vi "ADC_Driver.vi"() -> ()   [LabVIEW 2020]
uses:
  <vilib>/numeric/Random Number (Range) DBL.vi
panel:
  out "Digital Waveform Graph":digitaldata(graph)
  out "Output Waveform":digitaldata
  out "x-y":u8[](array[numeric])
  out "Waveform Graph":u8[](graph)
  out "Unsigned Byte Array":u8[](array[numeric])
  out "Binary String":string
  out "Digital before U8":dbl
  in  "No of Bits":i32=2
  in  "Vref":dbl=5.0
  out "Analog ip":dbl
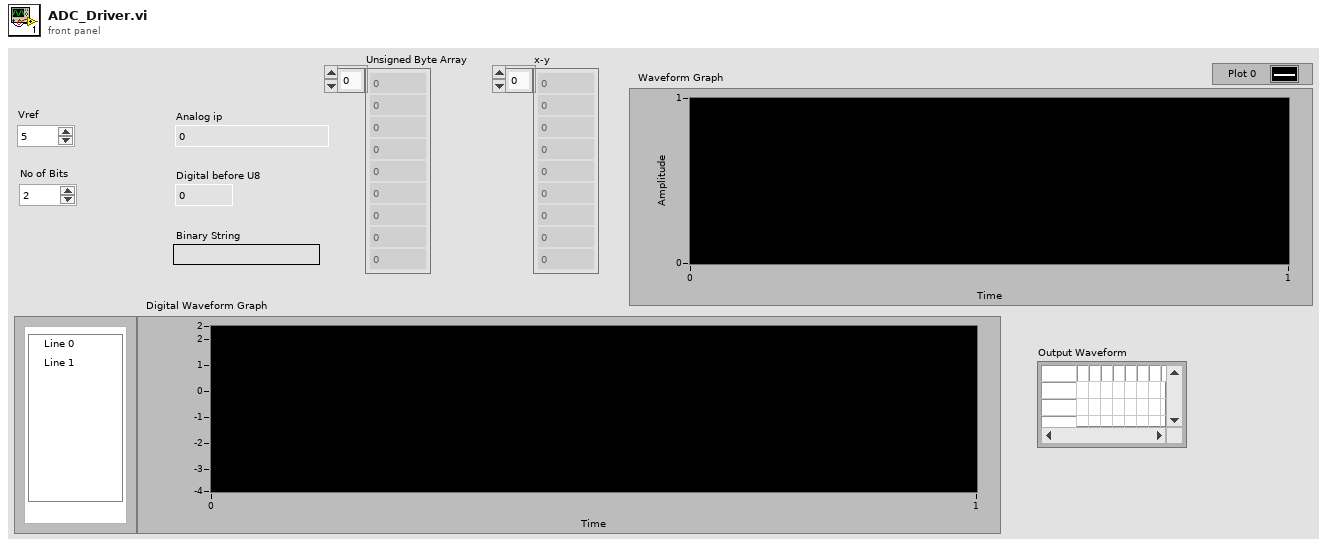
[diagram p1: front panel]
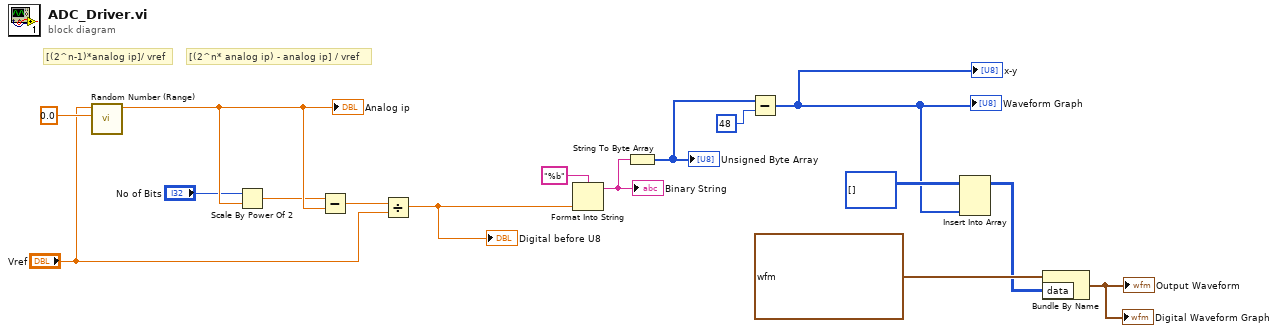
[diagram p0: block diagram]
diagram:
  # "[(2^n* analog ip) - analog ip] / vref"
  # "[(2^n-1)*analog ip]/ vref"
  n1 = call-poly <vilib>:"Random Number (Range).vi"("lower bound (0)"=0.0, "upper bound (100)"="Vref") -> ("number"=w15:dbl)  [unwired: 9 in]
  "Analog ip" <- w15
  n2 = Scale By Power Of 2(n="No of Bits", x=w15) -> (x*2^n=w14:dbl)
  n3 = Subtract(x=w14, y=w15) -> (x-y=w6:dbl)
  n4 = Divide(x=w6, y="Vref") -> (x/y=w12:dbl)
  "Digital before U8" <- w12
  n5 = Format Into String(format string="%b", w12) -> (resulting string=w10:string)  [unwired: 2 in, 1 out]
  "Binary String" <- w10
  n6 = String To Byte Array(string=w10) -> (unsigned byte array=w8:u8[])
  "Unsigned Byte Array" <- w8
  n7 = Subtract(x=w8, y=u8 48) -> (x-y=w3:u8[])
  "Waveform Graph" <- w3
  "x-y" <- w3
  n8 = Insert Into Array(array=i32[][] [], new element=w3) -> (w2:i32[][])  [unwired: 2 in]
  n9 = Bundle By Name(cluster=digitaldata {"transitions"=[], "data"=[]} ("waveform"), "data"=w2) -> (→"Output Waveform" →"Digital Waveform Graph":digitaldata)
